vi "Get_Parent_Children.vi"(10 "ID String":string, 11 "Map":map{string, cluster{string, variant}}(c390)) -> (0 "Class Name":string, 1 "Children":string[](array[string]), 2 "Found":bool, 3 "No Children":bool)   [LabVIEW 2025]
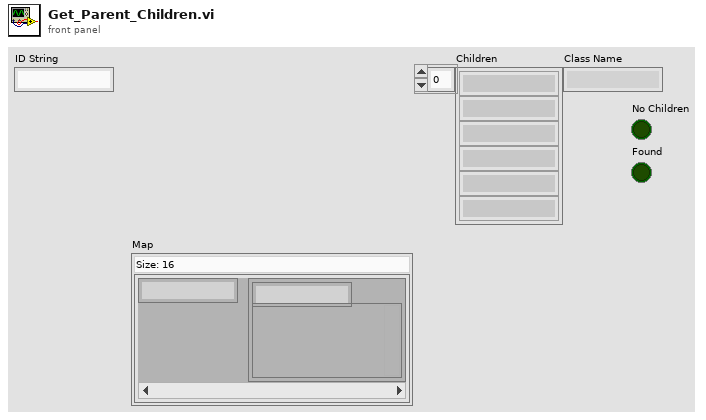
[diagram p1: front panel]
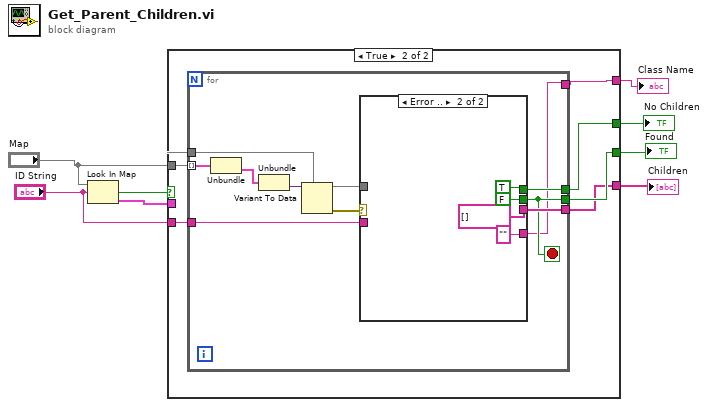
[diagram p0: block diagram]
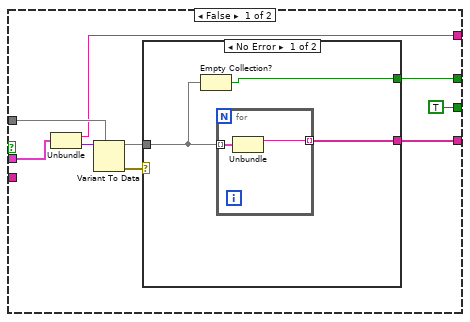
[diagram p2: hidden frame]
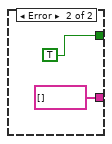
[diagram p3: hidden frame]
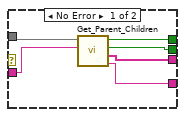
[diagram p4: hidden frame]
diagram:
  n1 = Look In Map(map="Map", key="ID String") -> (key not found?=w7:bool, value=w6:cluster{string, variant})  [unwired: 1 in]
  n2 = case shown="True" w7 {
    tunnel: "Map" -> [w15 w30]
    tunnel: w6 -> [w16 _]
    tunnel: [w13 w28] -> w5
    tunnel: [w11 w26] -> w4
    tunnel: [TRUE w27] -> w3
    tunnel: "ID String" -> [_ w29]
    tunnel: [w9 w25] -> w1
    frame False {
      n3 = Unbundle(w16) -> (w9:string, w17:variant)
      n4 = Variant To Data(type=w15, Variant=w17) -> (data=w12:map{string, cluster{string, variant}}, error out=w14:errorcluster)  [unwired: 1 in]
      n5 = case shown="No Error" w14 {
        tunnel: [w18 TRUE] -> w13
        tunnel: w12 -> [w19 _]
        tunnel: [w20 string[] []] -> w11
        frame No Error {
          n6 = Empty Collection?(1:w19) -> (0:w18:bool)
          n7 = for {
            tunnel: w19 -> [w22] mode=indexing
            tunnel: [w21] -> w20 mode=indexing
            n8 = Unbundle(w22) -> (w21:string)  [unwired: 1 out]
          }
        }
        frame Error {
        }
      }
    }
    frame True {
      n9 = for {
        tunnel: w30 -> [w41] mode=indexing
        tunnel: w30 -> [w38]
        tunnel: w29 -> [w35]
        tunnel: [w34] -> w28
        tunnel: [w32] -> w27
        tunnel: [w33] -> w26
        tunnel: [w31] -> w25
        stop <- w32 stop-if-true
        n10 = Unbundle(w41) -> (w40:cluster{string, variant})  [unwired: 1 out]
        n11 = Unbundle(w40) -> (w39:variant)  [unwired: 1 out]
        n12 = Variant To Data(type=w38, Variant=w39) -> (data=w36:map{string, cluster{string, variant}}, error out=w37:errorcluster)  [unwired: 1 in]
        n13 = case shown="Error .." w37 {
          tunnel: w36 -> [w47 _]
          tunnel: w35 -> [w46 _]
          tunnel: [w45 TRUE ("No Children")] -> w34
          tunnel: [w44 FALSE ("Found")] -> w32
          tunnel: [w43 string[] [] ("Children")] -> w33
          tunnel: [w42 "" ("Class Name")] -> w31
          frame No Error {
            n14 = call "Get_Parent_Children.vi"("ID String"=w46, "Map"=w47) -> ("Class Name"=w42:string, "Children"=w43:string[], "Found"=w44:bool, "No Children"=w45:bool)  [unwired: 6 in]
          }
          frame Error {
          }
        }
      }
    }
  }
  "No Children" <- w5
  "Children" <- w4
  "Found" <- w3
  "Class Name" <- w1
